vi "Flatness-SetupFrequency.vi"(0 "Session In":refnum<visa-resource-name>="TCPIP0::169.254.70.100::inst0::INSTR", 1 "Timeout":u32=3000, 5 "error in":errorcluster {"code" format="%.0x"}, 7 "Select":i32(ring) items=["START", "STOP", "POINTS"], 9 "Freq/poin":dbl=20000.0, 10 "RO(T)":bool, 11 "Units":u16(ring) items=["Hz", "MHz", "GHz"]) -> (12 "success?":bool, 14 "Session Out":refnum<visa-resource-name>, 19 "error out":errorcluster {"code" format="%.0x"})   [LabVIEW 2018]
doc: "Launches the Instrument I/O Assistant, which you can use to communicate with message-based instruments and graphically parse the response. For example you can communicate with an instrument that uses a serial, Ethernet, or GPIB interface."
uses:
  Agilent PSG MXG Series.lvlib
panel:
  out "read":dbl
  out "read(str)":string
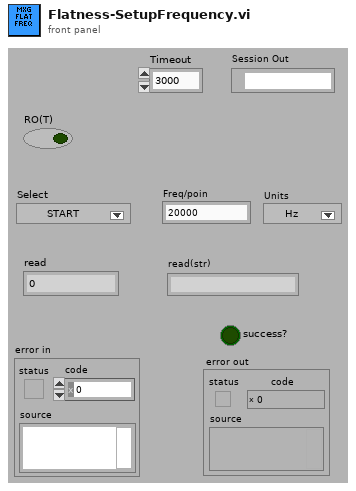
[diagram p1: front panel]
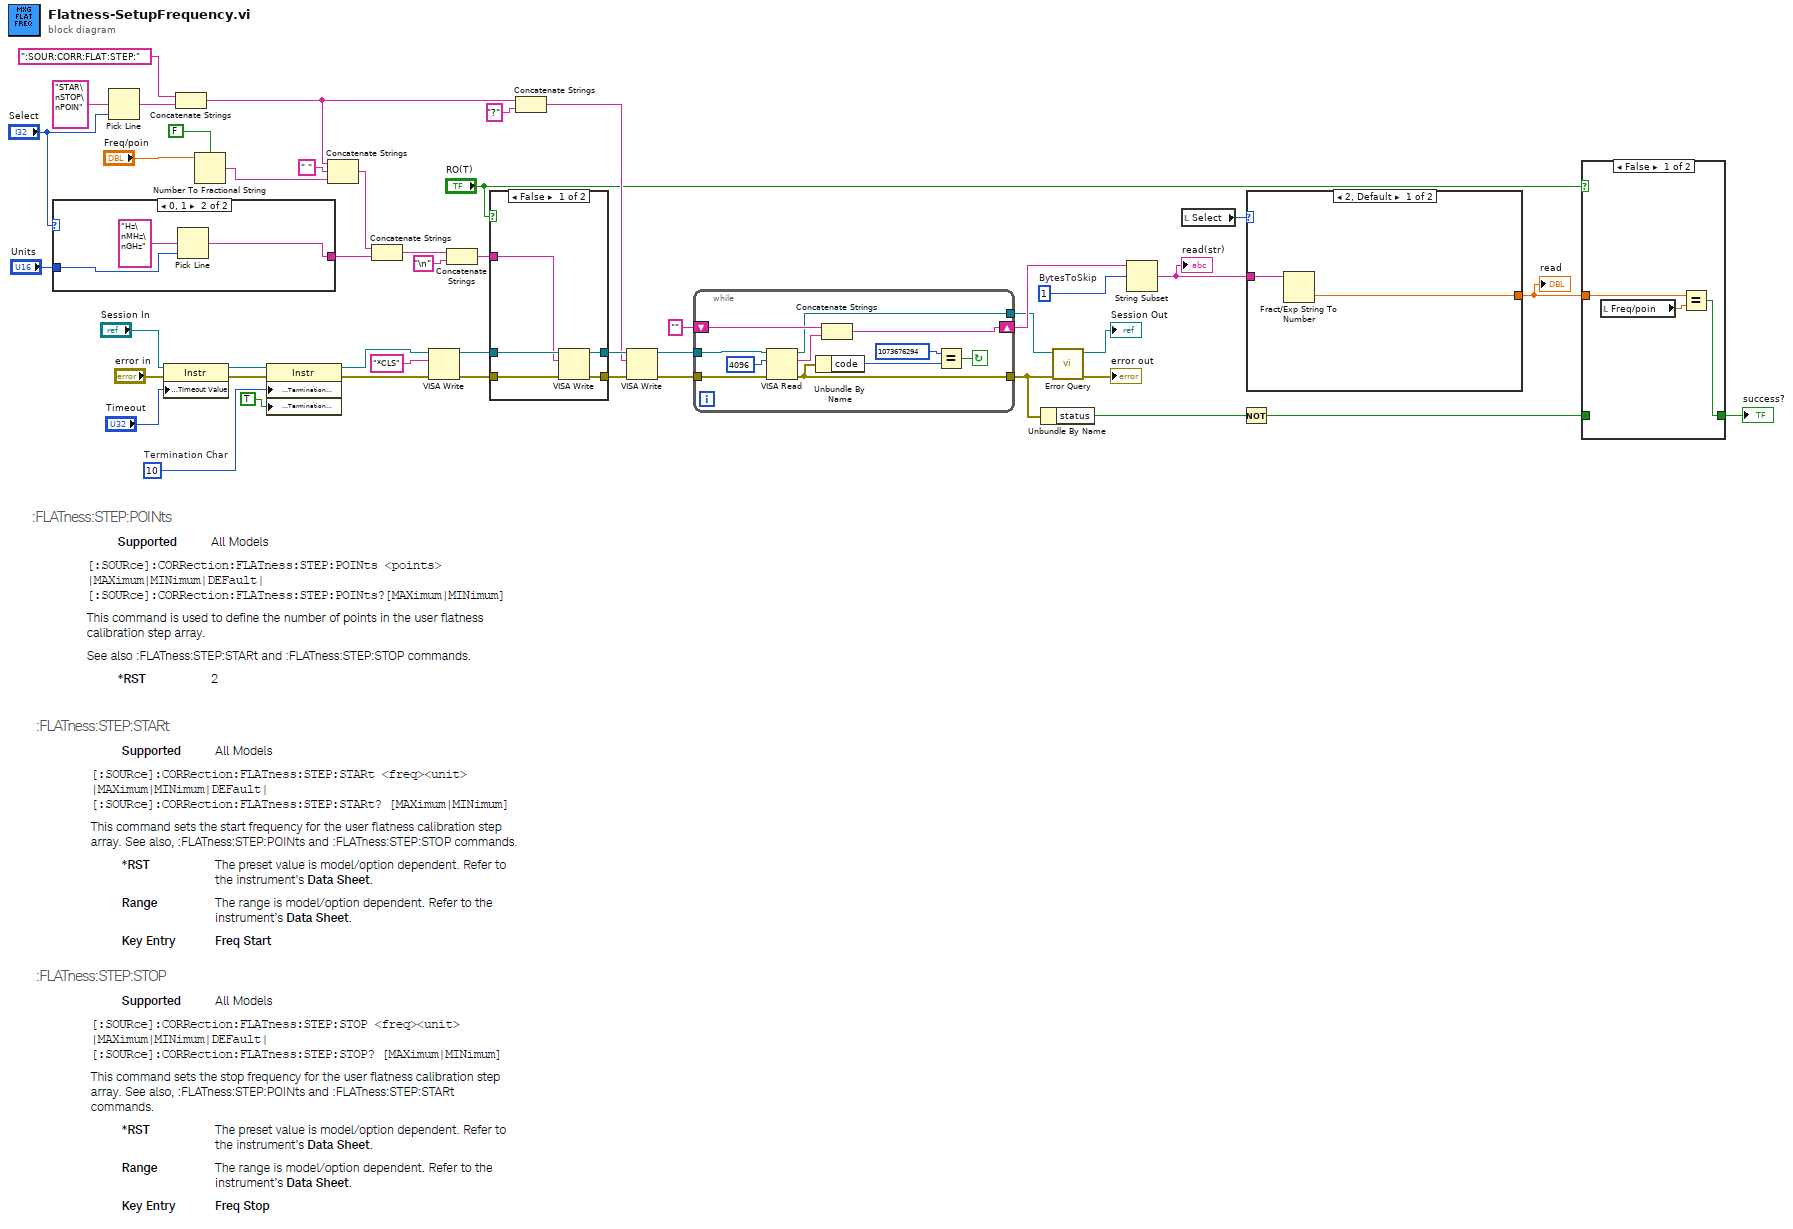
[diagram p0: block diagram]
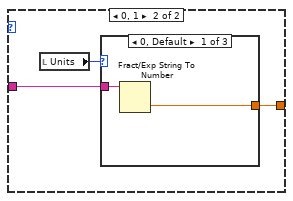
[diagram p2: hidden frame]
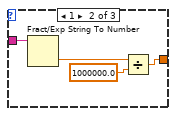
[diagram p3: hidden frame]
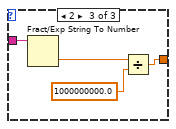
[diagram p4: hidden frame]
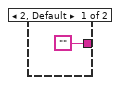
[diagram p6: hidden frame]
diagram:
  w35 = 1  # BytesToSkip
  w42 = u8 10  # Termination Char
  n1 = case shown="0, 1" "Select" {
    tunnel: "Units" -> [_ w50]
    tunnel: ["" w51] -> w18
    frame 2, Default {
    }
    frame 0, 1 {
      n2 = Pick Line(multi-line string="Hz\nMHz\nGHz", line index=w50) -> (output string=w51:string)  [unwired: 1 in]
    }
  }
  n3 = Pick Line(multi-line string="STAR\nSTOP\nPOIN", line index="Select") -> (output string=w20:string)  [unwired: 1 in]
  n4 = property class="Instr"(reference="Session In", error in="error in", "General Settings:Timeout Value"="Timeout") -> (reference out=w41:refnum<visa-resource-name>, error out=w43:errorcluster)
  n5 = Concatenate Strings(":SOUR:CORR:FLAT:STEP:" ("staticText"), w20) -> (w25:string)
  n6 = Number To Fractional String(use system decimal point (T)=FALSE, number="Freq/poin") -> (F-format string=w33:string)  [unwired: 2 in]
  n7 = property class="Instr"(reference=w41, error in=w43, "Message Based Settings:Termination Character"=w42, "Message Based Settings:Termination Character Enable"=TRUE ("enable")) -> (reference out=w3:refnum<visa-resource-name>, error out=w2:errorcluster)
  n8 = Concatenate Strings(w25, " " ("staticText"), w33) -> (w31:string)
  n9 = Concatenate Strings(w31, w18) -> (w30:string)
  n10 = VISA Write(VISA resource name=w3, write buffer="*CLS", error in (no error)=w2) -> (VISA resource name out=w4:refnum<visa-resource-name>, error out=w5:errorcluster)  [unwired: 1 out]
  n11 = Concatenate Strings(w30, "\n" ("StaticText")) -> (w26:string)
  n12 = case shown="False" "RO(T)" {
    tunnel: [w56 w57] -> w28
    tunnel: [w55 w58] -> w27
    tunnel: w4 -> [w54 w58]
    tunnel: w5 -> [w53 w57]
    tunnel: w26 -> [w52 _]
    frame False {
      n13 = VISA Write(VISA resource name=w54, write buffer=w52, error in (no error)=w53) -> (VISA resource name out=w55:refnum<visa-resource-name>, error out=w56:errorcluster)  [unwired: 1 out]
    }
    frame True {
    }
  }
  n14 = Concatenate Strings(w25, "?" ("string")) -> (w22:string)
  n15 = VISA Write(VISA resource name=w27, write buffer=w22, error in (no error)=w28) -> (VISA resource name out=w39:refnum<visa-resource-name>, error out=w38:errorcluster)  [unwired: 1 out]
  n16 = while {
    tunnel: w39 -> [w66]
    shift-right: [w60] -> w36
    shift-left: "" -> [w65]
    tunnel: w38 -> [w63]
    tunnel: [w62] -> w9
    tunnel: [w59] -> w8
    stop <- w61 continue-if-true
    n17 = VISA Read(VISA resource name=w66, byte count=u32 4096 ("byte count (0)"), error in (no error)=w63) -> (VISA resource name out=w59:refnum<visa-resource-name>, read buffer=w64:string, error out=w62:errorcluster)  [unwired: 1 out]
    n18 = Unbundle By Name(w62) -> ("code"=w68:i32)
    n19 = Concatenate Strings(w65, w64) -> (w60:string)
    n20 = Equal?(x=1073676294, y=w68) -> (x = y?=w61:bool)
  }
  n21 = Unbundle By Name(w9) -> ("status"=w13:bool)
  n22 = call "Error Query.vi"("error in (no error)"=w9, "VISA resource name"=w8) -> ("error out"=→"error out":errorcluster, "VISA resource name out"=→"Session Out":refnum<visa-resource-name>)  [unwired: 6 in, 2 out]
  n23 = String Subset(string=w36, offset (0)=w35) -> (substring=w23:string)  [unwired: 1 out]
  "read(str)" <- w23
  n24 = local read "Select"() -> (w11:i32)
  n25 = Not(x=w13) -> (.not. x?=w12:bool)
  n26 = case shown="2, Default" w11 {
    tunnel: w23 -> [w71 w74]
    tunnel: [w70 w73] -> w16
    frame 2, Default {
      n27 = Fract/Exp String To Number(string=w71) -> (number=w70:dbl)  [unwired: 3 in, 1 out]
    }
    frame 0, 1 {
      n28 = local read "Units"() -> (w72:u16)
      n29 = case shown="0, Default" w72 {
        tunnel: w74 -> [w76 w80 w84]
        tunnel: [w75 w79 w83] -> w73
        frame 0, Default {
          n30 = Fract/Exp String To Number(string=w76) -> (number=w75:dbl)  [unwired: 3 in, 1 out]
        }
        frame 1 {
          n31 = Fract/Exp String To Number(string=w80) -> (number=w78:dbl)  [unwired: 3 in, 1 out]
          n32 = Divide(x=w78, y=1000000.0) -> (x/y=w79:dbl)
        }
        frame 2 {
          n33 = Fract/Exp String To Number(string=w84) -> (number=w82:dbl)  [unwired: 3 in, 1 out]
          n34 = Divide(x=w82, y=1000000000.0) -> (x/y=w83:dbl)
        }
      }
    }
  }
  "read" <- w16
  n35 = case shown="False" "RO(T)" {
    tunnel: w16 -> [w87 _]
    tunnel: [w85 w88] -> w15
    tunnel: w12 -> [_ w88]
    frame False {
      n36 = local read "Freq/poin"() -> (w86:dbl)
      n37 = Equal?(x=w87, y=w86) -> (x = y?=w85:bool)
    }
    frame True {
    }
  }
  "success?" <- w15
